vi "过0法子程序.vi"(1 "波形":waveform(dbl)) -> (0 "f":dbl)   [LabVIEW 2017]
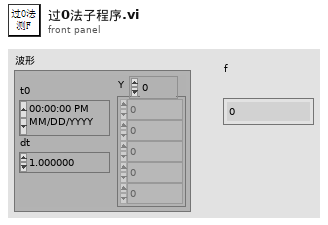
[diagram p1: front panel]
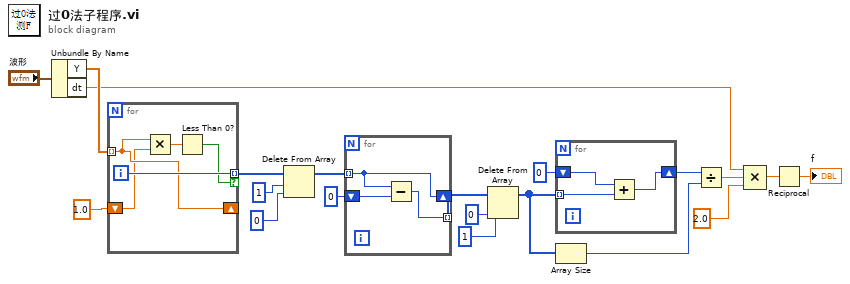
[diagram p0: block diagram]
diagram:
  n1 = Unbundle By Name("波形") -> ("Y"=w20:dbl[], "dt"=w6:dbl)
  n2 = for {
    tunnel: w20 -> [w22] mode=indexing
    shift-right: [w22] -> _
    shift-left: 1.0 -> [w21]
    tunnel: [w24] -> w18 mode=indexing if=w23
    i -> [w24]
    n3 = Multiply(x=w22, y=w21) -> (x*y=w25:dbl)
    n4 = Less Than 0?(x=w25) -> (x < 0?=w23:bool)
  }
  n5 = Delete From Array(array=w18, length=1 ("长度"), index=0 ("索引")) -> (array with subset deleted=w15:i32[])  [unwired: 1 out]
  n6 = for {
    tunnel: w15 -> [w27] mode=indexing
    shift-right: [w27] -> _
    shift-left: 0 -> [w28]
    tunnel: [w26] -> w11 mode=indexing
    n7 = Subtract(x=w27, y=w28) -> (x-y=w26:i32)
  }
  n8 = Delete From Array(array=w11, length=1 ("长度"), index=0 ("索引")) -> (array with subset deleted=w8:i32[])  [unwired: 1 out]
  n9 = for {
    tunnel: w8 -> [w30] mode=indexing
    shift-right: [w29] -> w9
    shift-left: 0 -> [w31]
    n10 = Add(x=w31, y=w30) -> (x+y=w29:i32)
  }
  n11 = Array Size(array=w8) -> (size(s)=w7:i32)
  n12 = Divide(x=w9, y=w7) -> (x/y=w5:dbl)
  n13 = Compound Arithmetic op=MULTIPLY(w6, w5, 2.0 ("值")) -> (w3:dbl)
  n14 = Reciprocal(x=w3) -> (1/x=→"f":dbl)
